vi "ImaqToPic.vi"(7 "Image Src":T1) -> (0 "error out":errorcluster, 3 "picture":picture)   [LabVIEW 2011]
uses:
  <vilib>/vision/Image Controls.llb/IMAQ Image.ctl
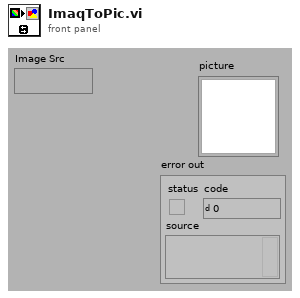
[diagram p1: front panel]
types:
  T1 = typedef "IMAQ Image.ctl" = refnum<image>
  T2 = typedef "imagedata.ctl" = cluster{"image type":i32, "image depth":i32, "image":u8[], "mask":u8[], "colors":u32[], "Rectangle":cluster{"left":i16, "top":i16, "right":i16, "bottom":i16}}
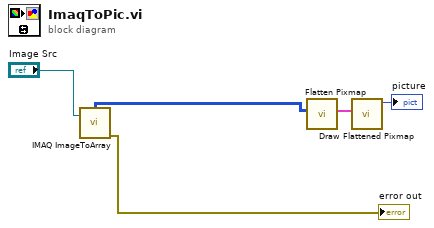
[diagram p0: block diagram]
diagram:
  n1 = call "IMAQ ImageToArray"("Image"="Image Src") -> ("error out"=→"error out":errorcluster, "Image Pixels (U8)"=w1:u8[][])  [unwired: 3 in, 3 out]
  n2 = call <vilib>:"Flatten Pixmap.vi"("8-bit pixmap"=w1) -> ("image data"=w5:T2)  [unwired: 10 in]
  n3 = call <vilib>:"Draw Flattened Pixmap.vi"("image data"=w5) -> ("new picture"=→"picture":picture)  [unwired: 8 in]
